vi "Close Notifiers.vi"(8 "error constant":errorcluster, 11 "output cluster":T1) -> (0 "error out":errorcluster)   [LabVIEW 2017]
uses:
  Notifiers.ctl
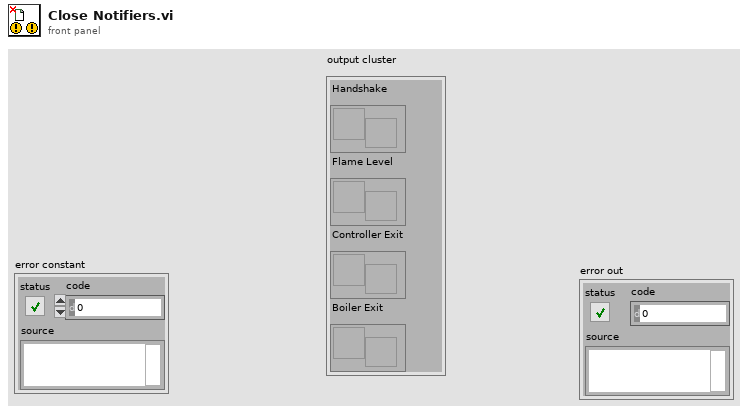
[diagram p1: front panel]
types:
  T1 = typedef "Notifiers.ctl" = cluster{"Handshake":refnum<notifier>, "Flame Level":refnum<notifier>, "Controller Exit":refnum<notifier>, "Boiler Exit":refnum<notifier>}
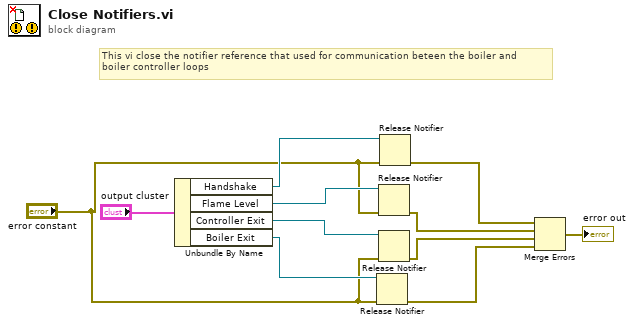
[diagram p0: block diagram]
diagram:
  # "This vi close the notifier reference that used for communication beteen the boiler and\nboiler controller loops"
  n1 = Unbundle By Name("output cluster") -> ("Handshake"=w9:refnum<notifier>, "Flame Level"=w8:refnum<notifier>, "Controller Exit"=w7:refnum<notifier>, "Boiler Exit"=w6:refnum<notifier>)
  n2 = Release Notifier(notifier=w6, error in (no error)="error constant") -> (error out=w1:errorcluster)  [unwired: 1 in, 2 out]
  n3 = Release Notifier(notifier=w8, error in (no error)="error constant") -> (error out=w3:errorcluster)  [unwired: 1 in, 2 out]
  n4 = Release Notifier(notifier=w7, error in (no error)="error constant") -> (error out=w2:errorcluster)  [unwired: 1 in, 2 out]
  n5 = Release Notifier(notifier=w9, error in (no error)="error constant") -> (error out=w4:errorcluster)  [unwired: 1 in, 2 out]
  n6 = Merge Errors(w4, w3, w2, w1) -> (→"error out":errorcluster)
